vi "Illini Hyperloop GUI v3.vi"() -> ()   [LabVIEW 2015]
uses:
  <vilib>/robotics/Controls/Attitude Indicator/Attitude Indicator.xctl
  <vilib>/ErrorRing/Error Ring.xnode
panel:
  out "Braking Force":dbl
  out "Braking Force Chart":dbl(slide) caption="Braking Force (N)" scale=0.0..10000.0
  out "Current 6":dbl[unit] caption="Current"
  out "Voltage 6":dbl[unit] caption="Voltage"
  out "RPM 6":dbl[unit] caption="RPM"
  out "Current 5":dbl[unit] caption="Current"
  out "Voltage 5":dbl[unit] caption="Voltage"
  out "RPM 5":dbl[unit] caption="RPM"
  out "Current 4":dbl[unit] caption="Current"
  out "Voltage 4":dbl[unit] caption="Voltage"
  out "RPM 4":dbl[unit] caption="RPM"
  out "Current 3":dbl[unit] caption="Current"
  out "Voltage 3":dbl[unit] caption="Voltage"
  out "RPM 3":dbl[unit] caption="RPM"
  out "Current 2":dbl[unit] caption="Current"
  out "Voltage 2":dbl[unit] caption="Voltage"
  out "RPM 2":dbl[unit] caption="RPM"
  out "Current 1":dbl[unit] caption="Current"
  out "Voltage 1":dbl[unit] caption="Voltage"
  out "RPM 1":dbl[unit] caption="RPM"
  out "Flight Time":string
  out "Attitude Indicator":cluster{"Roll":dbl, "Pitch":dbl}(xcontrol)
  out "Yaw":dbl(knob) scale=-20.0..20.0
  out "Gauge 6":dbl(knob) scale=0.0..2000.0
  out "Gauge 5":dbl(knob) scale=0.0..2000.0
  out "Gauge 4":dbl(knob) scale=0.0..2000.0
  out "Gauge 3":dbl(knob) scale=0.0..2000.0
  out "Gauge 2":dbl(knob) scale=0.0..2000.0
  out "Gauge":dbl(knob) scale=0.0..2000.0
  out "Cabin Pressure":dbl format="%#.3g"
  out "Cabin Pressure (psi)":dbl(graph)
  out "Stage":T1(ring)
  out "Communication Status":T2(ring)
  out "Levitation Height":dbl[unit]
  out "Computing:":dbl format="%#.2g"
  out "Low Battery":dbl format="%#.2g"
  out "High Battery:":dbl format="%#.2g"
  out "Battery 3":dbl(slide) scale=0.0..100.0
  out "Battery 2":dbl(slide) scale=0.0..100.0
  out "Battery 1":dbl(slide) scale=0.0..100.0
  out "Z acceleration":dbl
  out "Y acceleration":dbl
  out "X acceleration":dbl
  out "Z velocity":dbl
  out "Y velocity":dbl
  out "X velocity":dbl
  out "Z position":dbl
  out "Y position":dbl
  out "X position":dbl
  out "Position (m)":dbl(slide) scale=0.0..2490.0
  out "Checkmark":u16(ring)
  out "Velocity (m/s)":dbl(graph)
  in  "EMERGENCY BRAKE":bool
  in  "Functional Test Tab Control":T3(tab)
  out "Functional Test A Data":string caption="Data:"
  in  "Functional Test 1":bool caption="Boolean"
  out "Functional Test B Data":string caption="Data:"
  in  "Functional Test 2":bool caption="Boolean"
  out "Functional Test C Data":string caption="Data:"
  in  "Functional Test 3":bool caption="Boolean"
  in  "Functional Test 4":bool caption="Boolean"
  out "Functional Test D Data":string caption="Data:"
  in  "Client Closed":string="The client VI closed the connection."
  out "Data out":string
  in  "Functional Test 5":bool caption="Boolean"
  out "Temp 2:":dbl format="%.2g"
  out "Temp 1:":dbl format="%.2g"
  out "Temperature (K)":dbl[](graph)
  out "Acceleration Chart":dbl(graph)
  # "Illini Hyperloop"
  # "Arx Pax"
  # "Front"
  # "Attitude"
  # "Acceleration (m/s/s)"
  # "Battery Levels (%)"
  # "More battery?????"
  # "Functional Test A: Power Up and Communication"
  # "Functional Test B: Levitation"
  # "Functional Test C: Communication Inside Tube"
  # "Functional Test D: Internal power and Levitation"
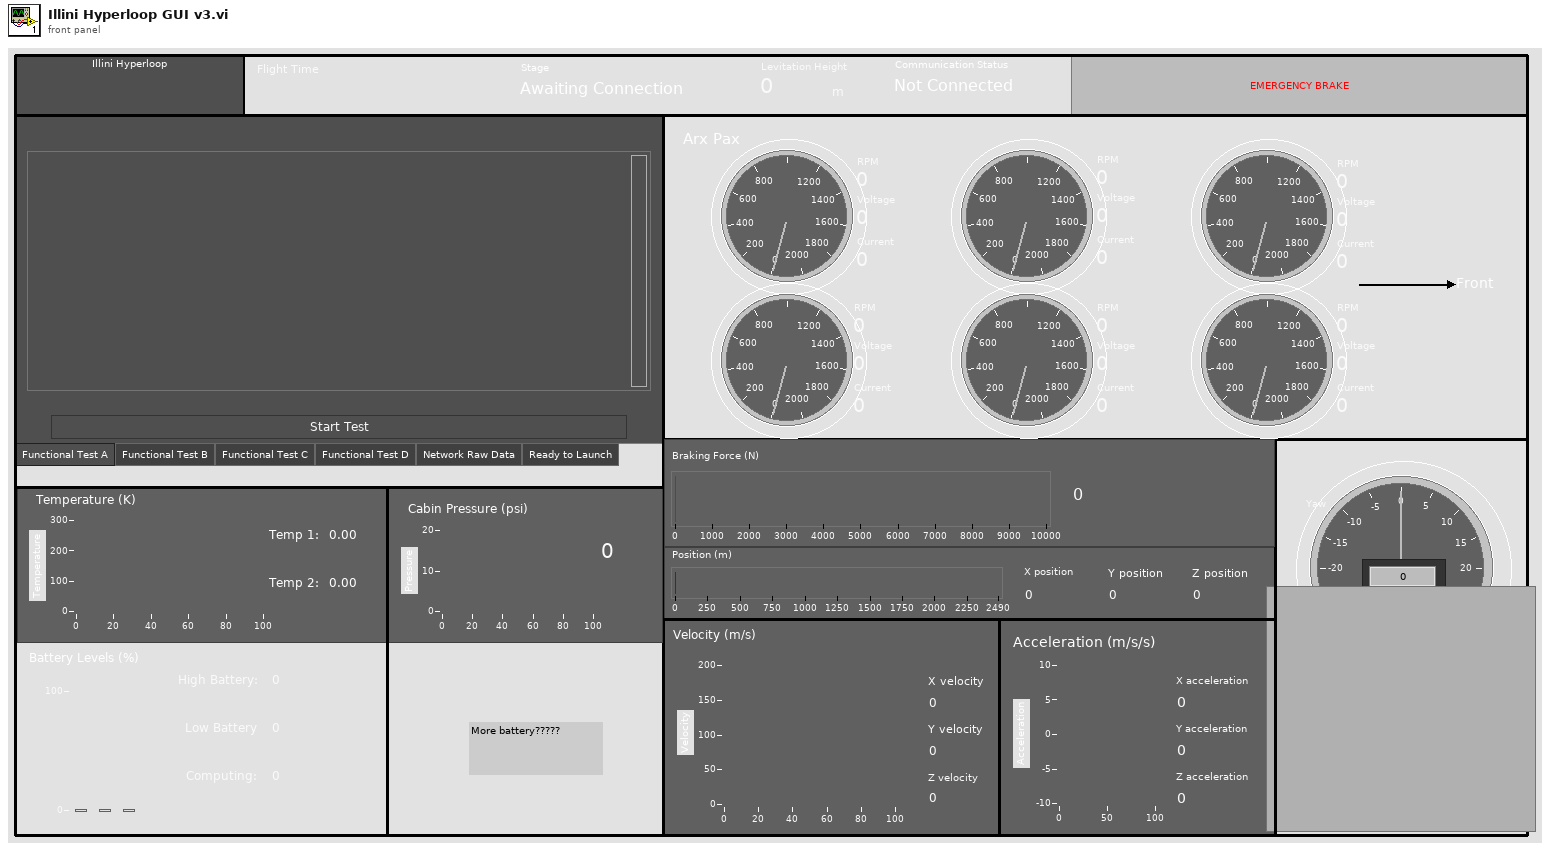
[diagram p1: front panel]
types:
  T1 = enum16{"Awaiting Connection", "TEST Comms", "TEST Lev", "TEST Inside Comms", "TEST Internal Power", "Ready to Launch", "Acceleration", "Coast", "Brake"}
  T2 = enum16{"Not Connected", "Connected", "Disconnected"}
  T3 = enum32{"Functional Test A", "Functional Test B", "Functional Test C", "Functional Test D", "Network Raw Data", "Ready to Launch"}
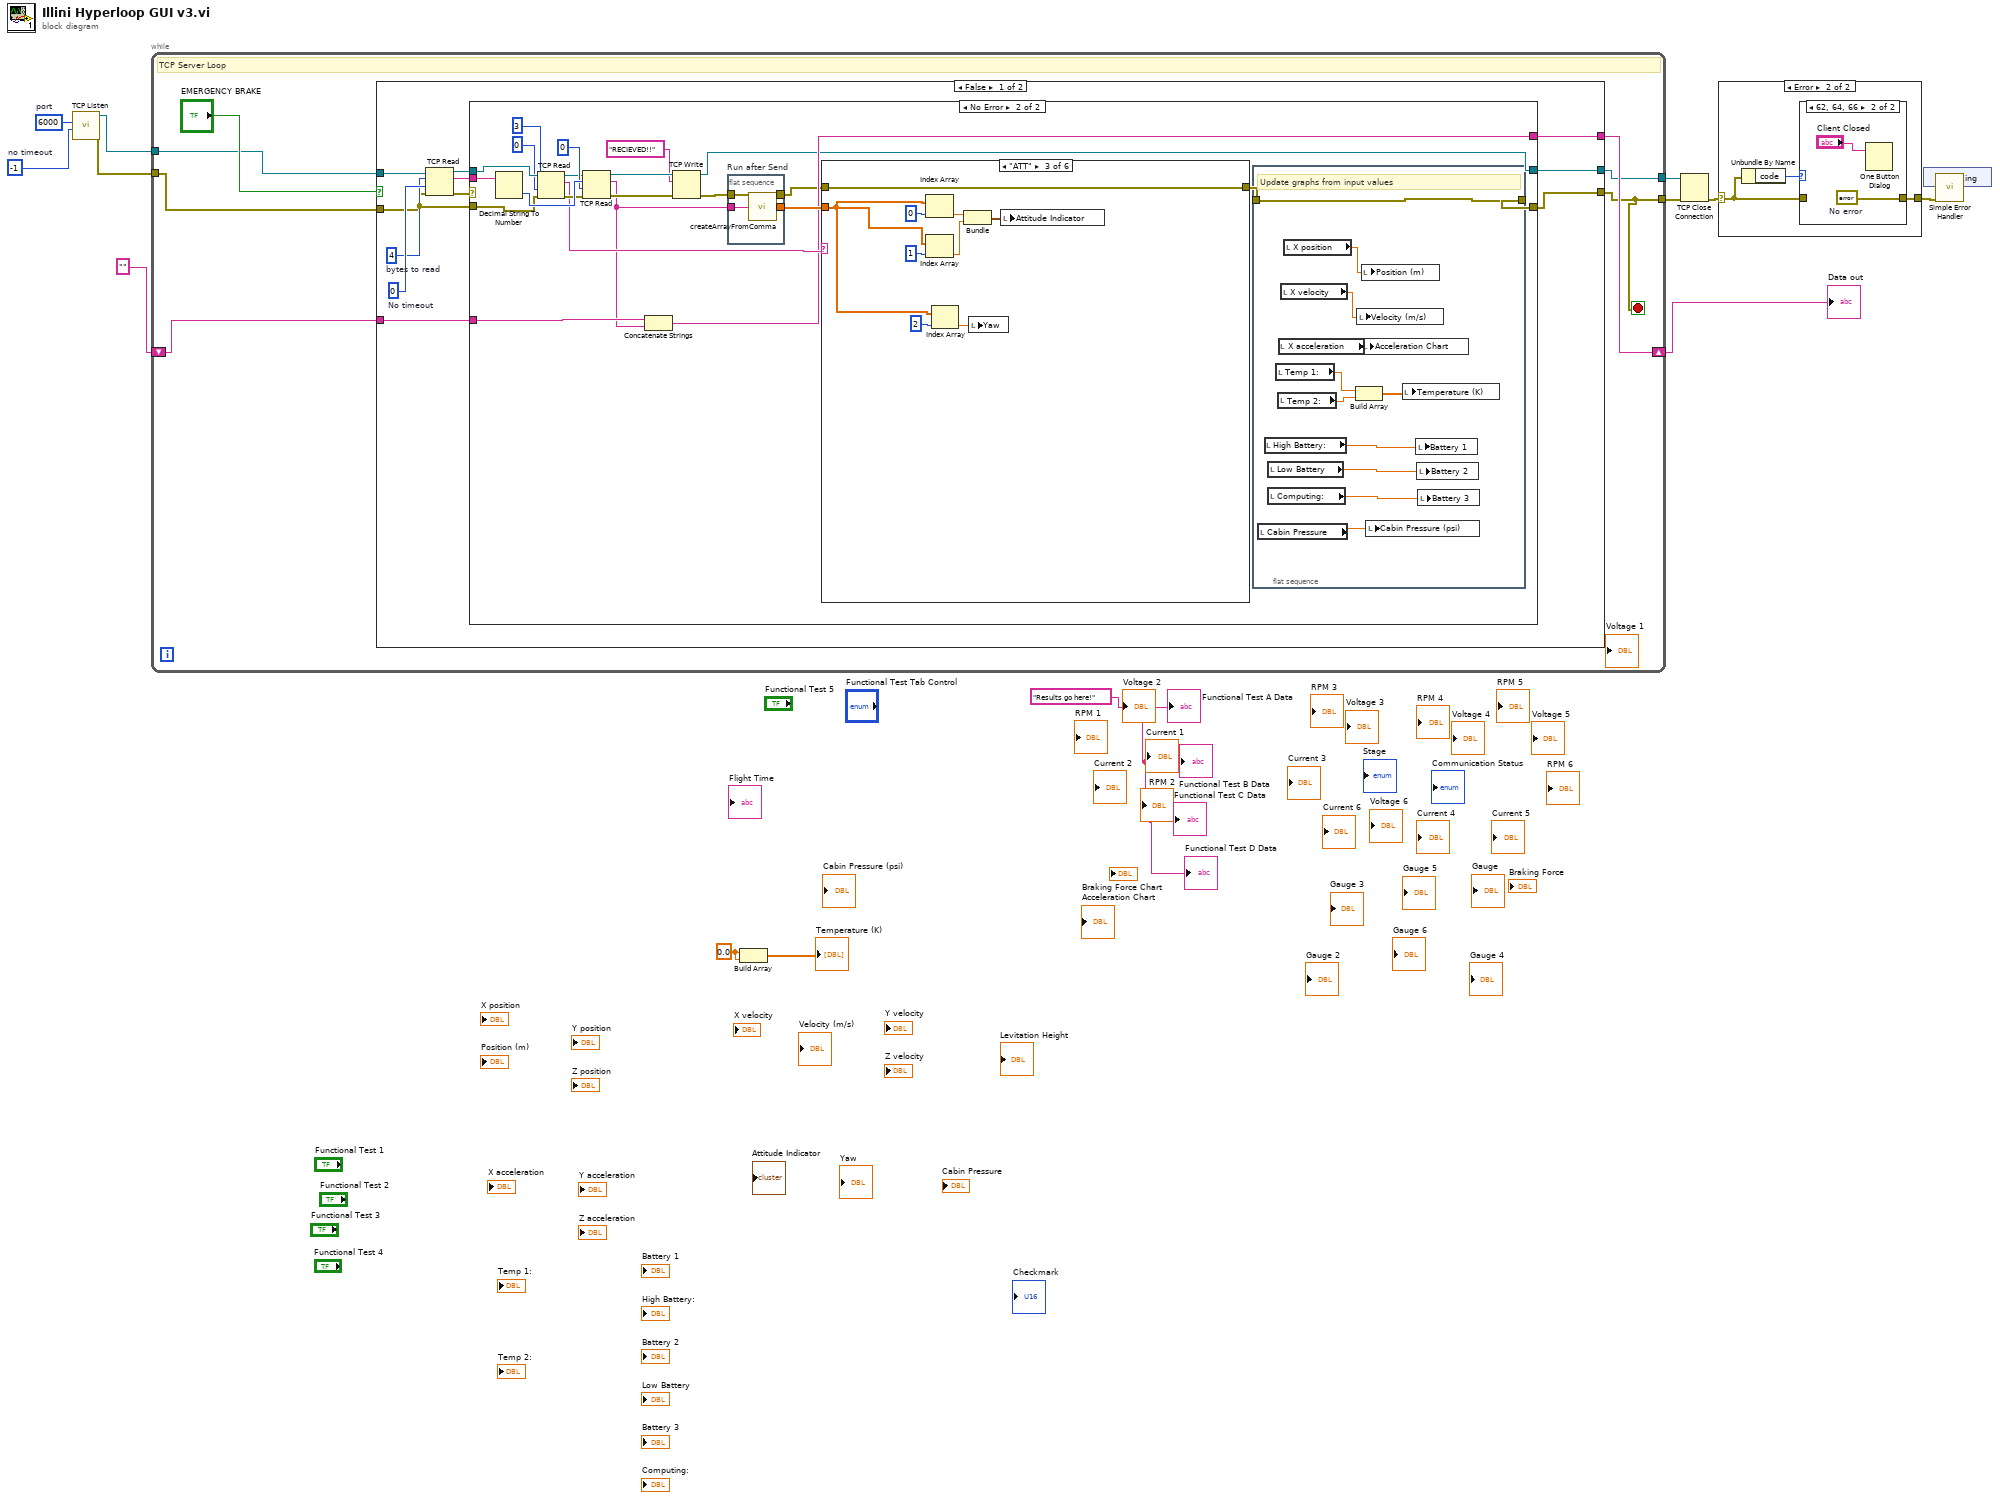
[diagram p0: block diagram]
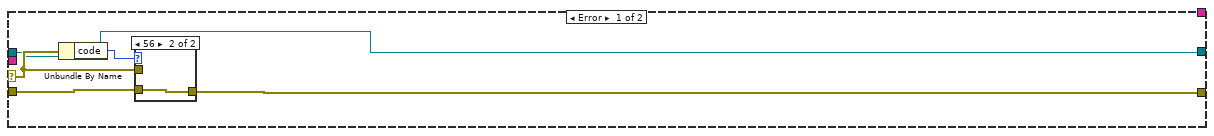
[diagram p4: hidden frame]
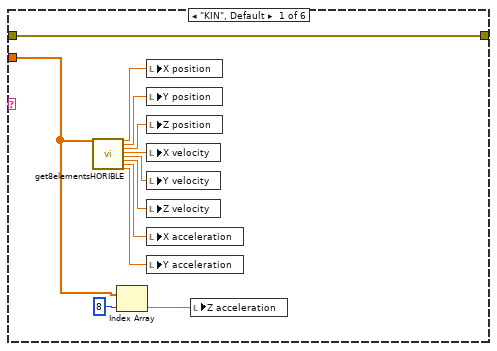
[diagram p6: hidden frame]
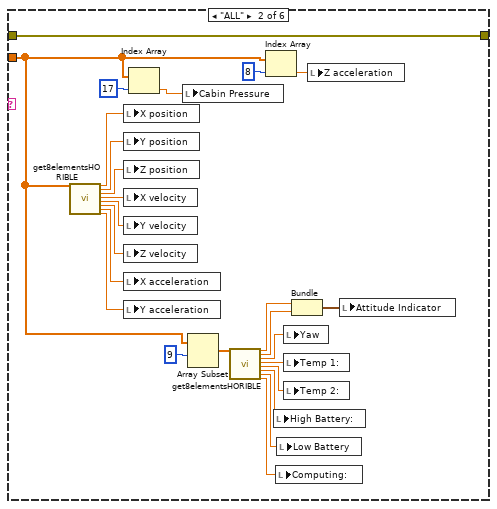
[diagram p7: hidden frame]
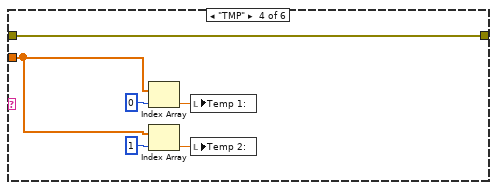
[diagram p8: hidden frame]
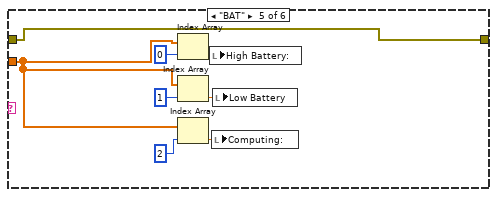
[diagram p9: hidden frame]
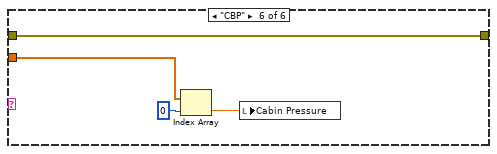
[diagram p10: hidden frame]
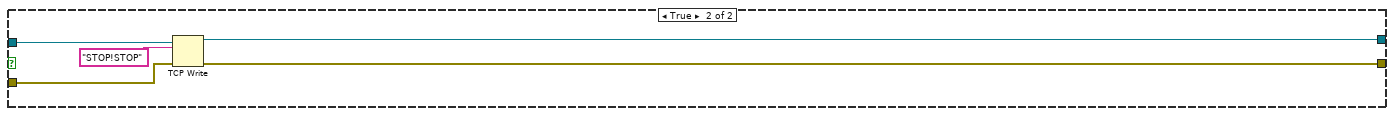
[diagram p11: hidden frame]
diagram:
  w1 = 0.0 ("element")
  w3 = "Results go here!" ("Functional Test 1 Data")
  w9 = u16 6000  # port
  w10 = -1  # no timeout
  n1 = call <vilib>:"TCP Listen.vi"("timeout ms (wait forever: -1)"=w10, "port"=w9) -> ("error out"=w11:errorcluster, "connection ID"=w6:refnum<k5>)  [unwired: 5 in, 3 out]
  n2 = while {
    tunnel: w6 -> [w18]
    tunnel: w11 -> [w19]
    shift-right: [w16] -> w7
    shift-left: "" -> [w17]
    tunnel: [w15] -> w5
    tunnel: [w14] -> w4
    stop <- w14 stop-if-true
    # "TCP Server Loop"
    n3 = case shown="False" "EMERGENCY BRAKE" {
      tunnel: w19 -> [w29 w143]
      tunnel: w18 -> [w30 w142]
      tunnel: [w25 w141] -> w15
      tunnel: [w27 w140] -> w14
      tunnel: w17 -> [w23 _]
      tunnel: [w22 _] -> w16
      frame False {
        w31 = 4  # bytes to read
        w32 = 0  # No timeout
        n4 = TCP Read(connection ID=w30, bytes to read=w31, error in (no error)=w29, 9:w32) -> (connection ID out=w26:refnum<k5>, data out=w24:string, error out=w28:errorcluster)  [unwired: 1 in]
        n5 = case shown="No Error" w28 {
          selector: w28 -> [w35 _]
          tunnel: w29 -> [w36 w54]
          tunnel: [w34 w47] -> w27
          tunnel: w26 -> [w33 w60]
          tunnel: [w33 w46] -> w25
          tunnel: w24 -> [_ w61]
          tunnel: w23 -> [_ w50]
          tunnel: [_ w49] -> w22
          frame Error {
            n6 = Unbundle By Name(w35) -> ("code"=w37:i32)
            n7 = case shown="56" w37 {
              tunnel: w35 -> [w38 _]
              tunnel: [w38 w39] -> w34
              tunnel: w36 -> [_ w39]
              frame Default {
              }
              frame 56 {
              }
            }
          }
          frame No Error {
            n8 = Decimal String To Number(string=w61) -> (number=w57:i32)  [unwired: 2 in, 1 out]
            n9 = TCP Read(connection ID=w60, bytes to read=3, error in (no error)=w54, 9:0 ("timeout ms (25000)")) -> (connection ID out=w55:refnum<k5>, data out=w52:string, error out=w53:errorcluster)  [unwired: 1 in]
            n10 = TCP Read(connection ID=w55, bytes to read=w57, error in (no error)=w53, 9:0 ("timeout ms (25000)")) -> (connection ID out=w45:refnum<k5>, data out=w42:string, error out=w43:errorcluster)  [unwired: 1 in]
            n11 = Concatenate Strings(w50, w42) -> (w49:string)
            n12 = TCP Write(connection ID=w45, data in="RECIEVED!!", error in (no error)=w43) -> (connection ID out=w46:refnum<k5>, error out=w41:errorcluster)  [unwired: 1 in, 1 out]
            n13 = flat-sequence "Run after Send" {
              tunnel: [w64] -> w51
              tunnel: w42 -> [w63]
              tunnel: w41 -> [w62]
              tunnel: [w62] -> w40
              frame #0 {
                n14 = call "createArrayFromComma.vi"("String"=w63) -> ("Array"=w64:dbl[])
              }
            }
            n15 = case shown="\"ATT\"" w52 {
              tunnel: w51 -> [w86 w90 w118 w125 w132 w138]
              tunnel: w40 -> [w84 w88 w113 w122 w128 w136]
              tunnel: [w84 w88 w113 w122 w128 w136] -> w48
              frame "KIN", Default {
                n16 = call "get8elementsHORIBLE.vi"("Array"=w86) -> ("Numeric"=w83:dbl, "Numeric 2"=w82:dbl, "Numeric 3"=w81:dbl, "Numeric 4"=w80:dbl, "Numeric 5"=w79:dbl, "Numeric 6"=w78:dbl, "Numeric 7"=w77:dbl, "Numeric 8"=w76:dbl)  [unwired: 19 in]
                n17 = Index Array(array=w86, index=8) -> (element=w85:dbl)
                n18 = local write "X position"(w83) -> ()
                n19 = local write "Y position"(w82) -> ()
                n20 = local write "Z position"(w81) -> ()
                n21 = local write "X velocity"(w80) -> ()
                n22 = local write "Y velocity"(w79) -> ()
                n23 = local write "Z velocity"(w78) -> ()
                n24 = local write "X acceleration"(w77) -> ()
                n25 = local write "Y acceleration"(w76) -> ()
                n26 = local write "Z acceleration"(w85) -> ()
              }
              frame "ALL" {
                n27 = call "get8elementsHORIBLE.vi"("Array"=w90) -> ("Numeric"=w110:dbl, "Numeric 2"=w109:dbl, "Numeric 3"=w108:dbl, "Numeric 4"=w107:dbl, "Numeric 5"=w106:dbl, "Numeric 6"=w105:dbl, "Numeric 7"=w104:dbl, "Numeric 8"=w103:dbl)  [unwired: 19 in]
                n28 = local write "X position"(w110) -> ()
                n29 = local write "Y position"(w109) -> ()
                n30 = local write "Z position"(w108) -> ()
                n31 = local write "X velocity"(w107) -> ()
                n32 = local write "Y velocity"(w106) -> ()
                n33 = local write "Z velocity"(w105) -> ()
                n34 = local write "X acceleration"(w104) -> ()
                n35 = local write "Y acceleration"(w103) -> ()
                n36 = Index Array(array=w90, index=17) -> (element=w89:dbl)
                n37 = local write "Cabin Pressure"(w89) -> ()
                n38 = Array Subset(array=w90, index=9) -> (w100:dbl[])  [unwired: 1 in]
                n39 = call "get8elementsHORIBLE.vi"("Array"=w100) -> ("Numeric"=w99:dbl, "Numeric 2"=w98:dbl, "Numeric 3"=w97:dbl, "Numeric 4"=w96:dbl, "Numeric 5"=w95:dbl, "Numeric 6"=w94:dbl, "Numeric 7"=w93:dbl, "Numeric 8"=w92:dbl)  [unwired: 19 in]
                n40 = Index Array(array=w90, index=8) -> (element=w111:dbl)
                n41 = local write "High Battery:"(w94) -> ()
                n42 = local write "Computing:"(w92) -> ()
                n43 = local write "Low Battery"(w93) -> ()
                n44 = local write "Yaw"(w97) -> ()
                n45 = local write "Temp 1:"(w96) -> ()
                n46 = local write "Temp 2:"(w95) -> ()
                n47 = Bundle("Numeric"=w99, "Numeric 2"=w98) -> (w102:cluster{"Numeric":dbl, "Numeric 2":dbl})  [unwired: 1 in]
                n48 = local write "Z acceleration"(w111) -> ()
                n49 = local write "Attitude Indicator"(w102) -> ()
              }
              frame "ATT" {
                n50 = Index Array(array=w118, index=0) -> (element=w117:dbl)
                n51 = Index Array(array=w118, index=1) -> (element=w116:dbl)
                n52 = Index Array(array=w118, index=2) -> (element=w114:dbl)
                n53 = Bundle(w117, w116) -> (w115:cluster{dbl, dbl})  [unwired: 1 in]
                n54 = local write "Yaw"(w114) -> ()
                n55 = local write "Attitude Indicator"(w115) -> ()
              }
              frame "TMP" {
                n56 = Index Array(array=w125, index=0) -> (element=w124:dbl)
                n57 = Index Array(array=w125, index=1) -> (element=w123:dbl)
                n58 = local write "Temp 1:"(w124) -> ()
                n59 = local write "Temp 2:"(w123) -> ()
              }
              frame "BAT" {
                n60 = Index Array(array=w132, index=0) -> (element=w131:dbl)
                n61 = Index Array(array=w132, index=1) -> (element=w130:dbl)
                n62 = Index Array(array=w132, index=2) -> (element=w129:dbl)
                n63 = local write "High Battery:"(w131) -> ()
                n64 = local write "Computing:"(w129) -> ()
                n65 = local write "Low Battery"(w130) -> ()
              }
              frame "CBP" {
                n66 = Index Array(array=w138, index=0) -> (element=w137:dbl)
                n67 = local write "Cabin Pressure"(w137) -> ()
              }
            }
            n68 = flat-sequence {
              tunnel: w48 -> [w72]
              tunnel: [w72] -> w47
              frame #0 {
                # "Update graphs from input values"
                n69 = local read "Cabin Pressure"() -> (w68:dbl)
                n70 = local read "High Battery:"() -> (w71:dbl)
                n71 = local read "Low Battery"() -> (w70:dbl)
                n72 = local read "Computing:"() -> (w69:dbl)
                n73 = local read "Temp 1:"() -> (w67:dbl)
                n74 = local read "Temp 2:"() -> (w66:dbl)
                n75 = local read "X acceleration"() -> (w73:dbl)
                n76 = local read "X velocity"() -> (w74:dbl)
                n77 = local read "X position"() -> (w75:dbl)
                n78 = Build Array(w67, w66) -> (w65:dbl[])
                n79 = local write "Velocity (m/s)"(w74) -> ()
                n80 = local write "Acceleration Chart"(w73) -> ()
                n81 = local write "Position (m)"(w75) -> ()
                n82 = local write "Cabin Pressure (psi)"(w68) -> ()
                n83 = local write "Temperature (K)"(w65) -> ()
                n84 = local write "Battery 1"(w71) -> ()
                n85 = local write "Battery 2"(w70) -> ()
                n86 = local write "Battery 3"(w69) -> ()
              }
            }
          }
        }
      }
      frame True {
        n87 = TCP Write(connection ID=w142, data in="STOP!STOP", error in (no error)=w143) -> (connection ID out=w141:refnum<k5>, error out=w140:errorcluster)  [unwired: 1 in, 1 out]
      }
    }
    n88 = Wait (ms)(milliseconds to wait=u32 0) -> ()  [unwired: 1 out]
  }
  "Data out" <- w7
  n89 = Build Array(w1, w1) -> (→"Temperature (K)":dbl[])
  n90 = TCP Close Connection(connection ID=w5, error in (no error)=w4) -> (error out=w13:errorcluster)  [unwired: 2 out]
  n91 = case shown="Error" w13 {
    selector: w13 -> [w145 w147]
    tunnel: [w145 w146] -> w12
    frame No Error {
    }
    frame Error {
      n92 = Unbundle By Name(w147) -> ("code"=w148:i32)
      n93 = case shown="62, 64, 66" w148 {
        tunnel: w147 -> [w149 _]
        tunnel: [w149 w151] -> w146
        frame Default {
        }
        frame 62, 64, 66 {
          w151 = errorcluster {"status"=FALSE, "code"=0, "source"=""}  # No error
          n94 = One Button Dialog(message="Client Closed") -> ()  [unwired: 1 in, 1 out]
        }
      }
    }
  }
  n95 = xnode "Error Ring"() -> ()  [unwired: 1 out]
  n96 = call <vilib>:"Simple Error Handler.vi"("error in (no error)"=w12) -> ()  [unwired: 1 in, 8 out]
  "Functional Test A Data" <- w3
  "Functional Test B Data" <- w3
  "Functional Test C Data" <- w3
  "Functional Test D Data" <- w3
